vi "test.vi"() -> ()   [LabVIEW 2012]
uses:
  <vilib>/GPower/VIRegister/Library/Convert/ToStr.vi
  <vilib>/GPower/VIRegister/Library/SubVIs/FindRegisterData.vi
  <vilib>/GPower/VIRegister/Library/SubVIs/ReadSub.vi
  <vilib>/GPower/VIRegister/Library/QManager/GetRegisterData.vi
  <vilib>/GPower/Error/Library/SetError.vi
  <vilib>/GPower/Error/Library/FilterCodes.vi
  <vilib>/GPower/Error/Library/Filter/FilterMulti.vi
  <vilib>/GPower/VIRegister/Library/QManager/QManagerAction.vi
  <vilib>/GPower/Error/Library/ErrorType.vi
  <vilib>/GPower/Error/Library/SplitAppended.vi
  <vilib>/GPower/Error/Library/SubVIs/ExplanationToError.vi
  <vilib>/GPower/VIRegister/Library/QManager/GetQName.vi
  <vilib>/GPower/VIRegister/Library/QManager/StartQManager.vi
  <vilib>/Utility/error.llb/Trim Whitespace.vi
  <vilib>/dlg_ctls.llb/Space Constant.vi
  <vilib>/Utility/error.llb/Error Code Database.vi
  <vilib>/GPower/Error/Library/SubVIs/SetStatus.vi
  <vilib>/GPower/Error/Library/AppendErrors.vi
  <vilib>/GPower/Error/Library/Append/AppendSingle.vi
  <vilib>/GPower/VIRegister/VIRegister.lvlib
panel:
  out "Register value out":string
  in  "停止":bool
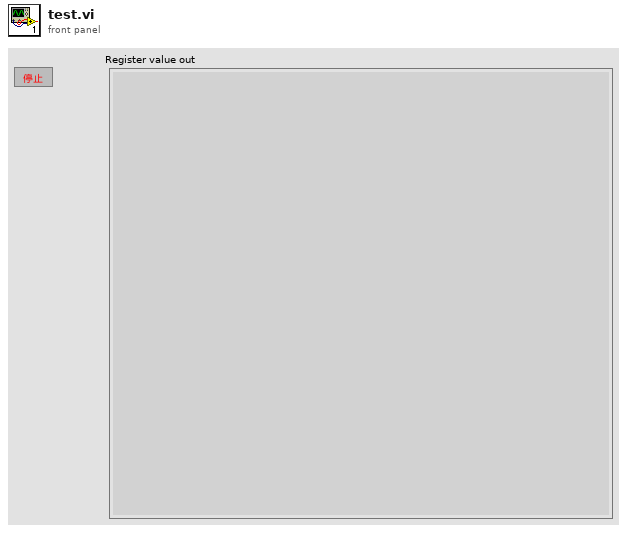
[diagram p1: front panel]
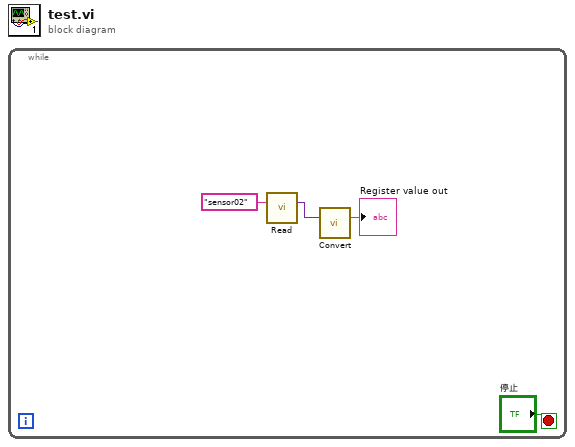
[diagram p0: block diagram]
diagram:
  n1 = while {
    stop <- "停止" stop-if-true
    n2 = call <vilib>:"Read.vi"("Register name"="sensor02") -> ("Register value"=w2:variant)  [unwired: 11 in, 3 out]
    n3 = call-poly <vilib>:"Convert.vi"("Register value in"=w2) -> ("Register value out"=→"Register value out":string)  [unwired: 13 in, 1 out]
  }
